vi "NodeSelected Event Callback.vi"(4 "NodeSelected":refnum<user-event>, 5 "事件数据":T1, 6 "控件引用":refnum<k24>, 7 "事件通用数据":cluster{"事件源":i32, "事件类型":u32, "时间标识":u32}) -> ()   [LabVIEW 2018]
uses:
  data/MyControlAll.dll
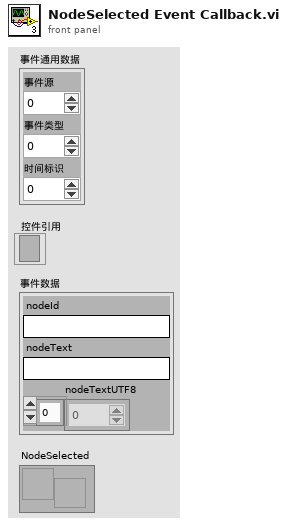
[diagram p1: front panel]
types:
  T1 = cluster{"nodeId":string, "nodeText":string, "nodeTextUTF8":u8[]}
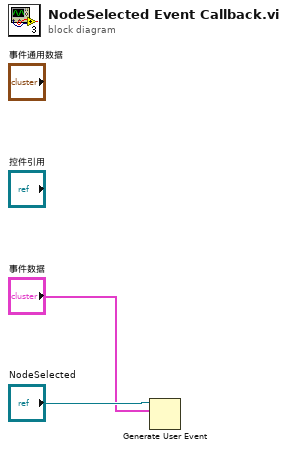
[diagram p0: block diagram]
diagram:
  n1 = Generate User Event(user event="NodeSelected", event data cluster="事件数据") -> ()  [unwired: 2 in, 2 out]
